vi "FlexRay_Table.vi"(8 "错误输入（无错误）":errorcluster, 9 "DataBase_array":refnum<vi>, 10 "FR_Buffer":T1[](array[typedef]), 11 "FlexRay_Data Ref":refnum<vi>) -> (0 "错误输出":errorcluster)   [LabVIEW 2014]
uses:
  Typedef/TLibFLexRay.ctl
  DataBase/Typedef/CAN/TCANSignal.ctl
  DataBase/Typedef/LIN/TLINSignal.ctl
  DataBase/Typedef/FlexRay/TFlexRaySignal.ctl
  DataBase/Typedef/TDBSignalProperties.ctl
  DataBase/Typedef/TDBFrameProperties.ctl
  DataBase/Typedef/TDBECUProperties.ctl
  DataBase/Typedef/TDBProperties.ctl
  DataBase/Typedef/DataBase_array.ctl
types:
  T1 = typedef "TLibFLexRay.ctl" = cluster{"FIdxChn":u8, "FChannelMask":u8, "FDir":u8, "FPayloadLength":u8, "FActualPayloadLength":u8, "FCycleNumber":u8, "FCCType":u8, "FFrameType":u8, "FHeaderCRCA":u16, "FHeaderCRCB":u16, "FFrameStateInfo":u16, "FSlotId":u16, "FFrameFlags":u32, "FFrameCRC":u32, "FReserved1":u64, "FReserved2":u64, "FTimeUs":u64, "FData":cluster{"数值":u8, "数值 9":u8, "数值 17":u8, "数值 25":u8, "数值 33":u8, "数值 41":u8, "数值 49":u8, "数值 57":u8, "数值 65":u8, "数值 73":u8, "数值 81":u8, "数值 89":u8, "数值 97":u8, "数值 105":u8, "数值 98":u8, "数值 99":u8, "数值 2":u8, "数值 10":u8, "数值 18":u8, "数值 26":u8, "数值 34":u8, "数值 42":u8, "数值 50":u8, "数值 58":u8, "数值 66":u8, "数值 74":u8, "数值 82":u8, "数值 90":u8, "数值 100":u8, "数值 106":u8, "数值 101":u8, "数值 102":u8, "数值 3":u8, "数值 11":u8, "数值 19":u8, "数值 27":u8, "数值 35":u8, "数值 43":u8, "数值 51":u8, "数值 59":u8, "数值 67":u8, "数值 75":u8, "数值 83":u8, "数值 91":u8, "数值 103":u8, "数值 107":u8, "数值 104":u8, "数值 108":u8, "数值 4":u8, "数值 12":u8, "数值 20":u8, "数值 28":u8, "数值 36":u8, "数值 44":u8, "数值 52":u8, "数值 60":u8, "数值 68":u8, "数值 76":u8, "数值 84":u8, "数值 92":u8, "数值 109":u8, "数值 110":u8, "数值 111":u8, "数值 112":u8, "数值 5":u8, "数值 13":u8, "数值 21":u8, "数值 29":u8, "数值 37":u8, "数值 45":u8, "数值 53":u8, "数值 61":u8, "数值 69":u8, "数值 77":u8, "数值 85":u8, "数值 93":u8, "数值 113":u8, "数值 114":u8, "数值 115":u8, "数值 116":u8, "数值 6":u8, "数值 14":u8, "数值 22":u8, "数值 30":u8, "数值 38":u8, "数值 46":u8, "数值 54":u8, "数值 62":u8, "数值 70":u8, "数值 78":u8, "数值 86":u8, "数值 94":u8, "数值 117":u8, "数值 118":u8, "数值 119":u8, "数值 120":u8, "数值 7":u8, "数值 15":u8, "数值 23":u8, "数值 31":u8, "数值 39":u8, "数值 47":u8, "数值 55":u8, "数值 63":u8, "数值 71":u8, "数值 79":u8, "数值 87":u8, "数值 95":u8, "数值 121":u8, "数值 122":u8, "数值 123":u8, "数值 124":u8, "数值 8":u8, "数值 16":u8, "数值 24":u8, "数值 32":u8, "数值 40":u8, "数值 48":u8, "数值 56":u8, "数值 64":u8, "数值 72":u8, "数值 80":u8, "数值 88":u8, "数值 96":u8, "数值 125":u8, "数值 126":u8, "数值 127":u8, "数值 128":u8, "数值 129":u8, "数值 130":u8, "数值 131":u8, "数值 132":u8, "数值 133":u8, "数值 134":u8, "数值 135":u8, "数值 136":u8, "数值 137":u8, "数值 138":u8, "数值 139":u8, "数值 140":u8, "数值 141":u8, "数值 142":u8, "数值 143":u8, "数值 144":u8, "数值 145":u8, "数值 146":u8, "数值 147":u8, "数值 148":u8, "数值 149":u8, "数值 150":u8, "数值 151":u8, "数值 152":u8, "数值 153":u8, "数值 154":u8, "数值 155":u8, "数值 156":u8, "数值 157":u8, "数值 158":u8, "数值 159":u8, "数值 160":u8, "数值 161":u8, "数值 162":u8, "数值 163":u8, "数值 164":u8, "数值 165":u8, "数值 166":u8, "数值 167":u8, "数值 168":u8, "数值 169":u8, "数值 170":u8, "数值 171":u8, "数值 172":u8, "数值 173":u8, "数值 174":u8, "数值 175":u8, "数值 176":u8, "数值 177":u8, "数值 178":u8, "数值 179":u8, "数值 180":u8, "数值 181":u8, "数值 182":u8, "数值 183":u8, "数值 184":u8, "数值 185":u8, "数值 186":u8, "数值 187":u8, "数值 188":u8, "数值 189":u8, "数值 190":u8, "数值 191":u8, "数值 192":u8, "数值 193":u8, "数值 194":u8, "数值 195":u8, "数值 196":u8, "数值 197":u8, "数值 198":u8, "数值 199":u8, "数值 200":u8, "数值 201":u8, "数值 202":u8, "数值 203":u8, "数值 204":u8, "数值 205":u8, "数值 206":u8, "数值 207":u8, "数值 208":u8, "数值 209":u8, "数值 210":u8, "数值 211":u8, "数值 212":u8, "数值 213":u8, "数值 214":u8, "数值 215":u8, "数值 216":u8, "数值 217":u8, "数值 218":u8, "数值 219":u8, "数值 220":u8, "数值 221":u8, "数值 222":u8, "数值 223":u8, "数值 224":u8, "数值 225":u8, "数值 226":u8, "数值 227":u8, "数值 228":u8, "数值 229":u8, "数值 230":u8, "数值 231":u8, "数值 232":u8, "数值 233":u8, "数值 234":u8, "数值 235":u8, "数值 236":u8, "数值 237":u8, "数值 238":u8, "数值 239":u8, "数值 241":u8, "数值 242":u8, "数值 243":u8, "数值 244":u8, "数值 245":u8, "数值 246":u8, "数值 247":u8, "数值 248":u8, "数值 249":u8, "数值 250":u8, "数值 251":u8, "数值 252":u8, "数值 253":u8, "数值 254":u8, "数值 255":u8}}
  T2 = cluster{"Message Name":string, "Signal Names":string[], "Signal_Values":dbl[]}
  T3 = cluster{"数值":u8, "数值 9":u8, "数值 17":u8, "数值 25":u8, "数值 33":u8, "数值 41":u8, "数值 49":u8, "数值 57":u8, "数值 65":u8, "数值 73":u8, "数值 81":u8, "数值 89":u8, "数值 97":u8, "数值 105":u8, "数值 98":u8, "数值 99":u8, "数值 2":u8, "数值 10":u8, "数值 18":u8, "数值 26":u8, "数值 34":u8, "数值 42":u8, "数值 50":u8, "数值 58":u8, "数值 66":u8, "数值 74":u8, "数值 82":u8, "数值 90":u8, "数值 100":u8, "数值 106":u8, "数值 101":u8, "数值 102":u8, "数值 3":u8, "数值 11":u8, "数值 19":u8, "数值 27":u8, "数值 35":u8, "数值 43":u8, "数值 51":u8, "数值 59":u8, "数值 67":u8, "数值 75":u8, "数值 83":u8, "数值 91":u8, "数值 103":u8, "数值 107":u8, "数值 104":u8, "数值 108":u8, "数值 4":u8, "数值 12":u8, "数值 20":u8, "数值 28":u8, "数值 36":u8, "数值 44":u8, "数值 52":u8, "数值 60":u8, "数值 68":u8, "数值 76":u8, "数值 84":u8, "数值 92":u8, "数值 109":u8, "数值 110":u8, "数值 111":u8, "数值 112":u8, "数值 5":u8, "数值 13":u8, "数值 21":u8, "数值 29":u8, "数值 37":u8, "数值 45":u8, "数值 53":u8, "数值 61":u8, "数值 69":u8, "数值 77":u8, "数值 85":u8, "数值 93":u8, "数值 113":u8, "数值 114":u8, "数值 115":u8, "数值 116":u8, "数值 6":u8, "数值 14":u8, "数值 22":u8, "数值 30":u8, "数值 38":u8, "数值 46":u8, "数值 54":u8, "数值 62":u8, "数值 70":u8, "数值 78":u8, "数值 86":u8, "数值 94":u8, "数值 117":u8, "数值 118":u8, "数值 119":u8, "数值 120":u8, "数值 7":u8, "数值 15":u8, "数值 23":u8, "数值 31":u8, "数值 39":u8, "数值 47":u8, "数值 55":u8, "数值 63":u8, "数值 71":u8, "数值 79":u8, "数值 87":u8, "数值 95":u8, "数值 121":u8, "数值 122":u8, "数值 123":u8, "数值 124":u8, "数值 8":u8, "数值 16":u8, "数值 24":u8, "数值 32":u8, "数值 40":u8, "数值 48":u8, "数值 56":u8, "数值 64":u8, "数值 72":u8, "数值 80":u8, "数值 88":u8, "数值 96":u8, "数值 125":u8, "数值 126":u8, "数值 127":u8, "数值 128":u8, "数值 129":u8, "数值 130":u8, "数值 131":u8, "数值 132":u8, "数值 133":u8, "数值 134":u8, "数值 135":u8, "数值 136":u8, "数值 137":u8, "数值 138":u8, "数值 139":u8, "数值 140":u8, "数值 141":u8, "数值 142":u8, "数值 143":u8, "数值 144":u8, "数值 145":u8, "数值 146":u8, "数值 147":u8, "数值 148":u8, "数值 149":u8, "数值 150":u8, "数值 151":u8, "数值 152":u8, "数值 153":u8, "数值 154":u8, "数值 155":u8, "数值 156":u8, "数值 157":u8, "数值 158":u8, "数值 159":u8, "数值 160":u8, "数值 161":u8, "数值 162":u8, "数值 163":u8, "数值 164":u8, "数值 165":u8, "数值 166":u8, "数值 167":u8, "数值 168":u8, "数值 169":u8, "数值 170":u8, "数值 171":u8, "数值 172":u8, "数值 173":u8, "数值 174":u8, "数值 175":u8, "数值 176":u8, "数值 177":u8, "数值 178":u8, "数值 179":u8, "数值 180":u8, "数值 181":u8, "数值 182":u8, "数值 183":u8, "数值 184":u8, "数值 185":u8, "数值 186":u8, "数值 187":u8, "数值 188":u8, "数值 189":u8, "数值 190":u8, "数值 191":u8, "数值 192":u8, "数值 193":u8, "数值 194":u8, "数值 195":u8, "数值 196":u8, "数值 197":u8, "数值 198":u8, "数值 199":u8, "数值 200":u8, "数值 201":u8, "数值 202":u8, "数值 203":u8, "数值 204":u8, "数值 205":u8, "数值 206":u8, "数值 207":u8, "数值 208":u8, "数值 209":u8, "数值 210":u8, "数值 211":u8, "数值 212":u8, "数值 213":u8, "数值 214":u8, "数值 215":u8, "数值 216":u8, "数值 217":u8, "数值 218":u8, "数值 219":u8, "数值 220":u8, "数值 221":u8, "数值 222":u8, "数值 223":u8, "数值 224":u8, "数值 225":u8, "数值 226":u8, "数值 227":u8, "数值 228":u8, "数值 229":u8, "数值 230":u8, "数值 231":u8, "数值 232":u8, "数值 233":u8, "数值 234":u8, "数值 235":u8, "数值 236":u8, "数值 237":u8, "数值 238":u8, "数值 239":u8, "数值 241":u8, "数值 242":u8, "数值 243":u8, "数值 244":u8, "数值 245":u8, "数值 246":u8, "数值 247":u8, "数值 248":u8, "数值 249":u8, "数值 250":u8, "数值 251":u8, "数值 252":u8, "数值 253":u8, "数值 254":u8, "数值 255":u8}
  T4 = typedef "LVRowAndColumnUnsignedTypeDef.ctl" = cluster{"Row":u32, "Column":u32}
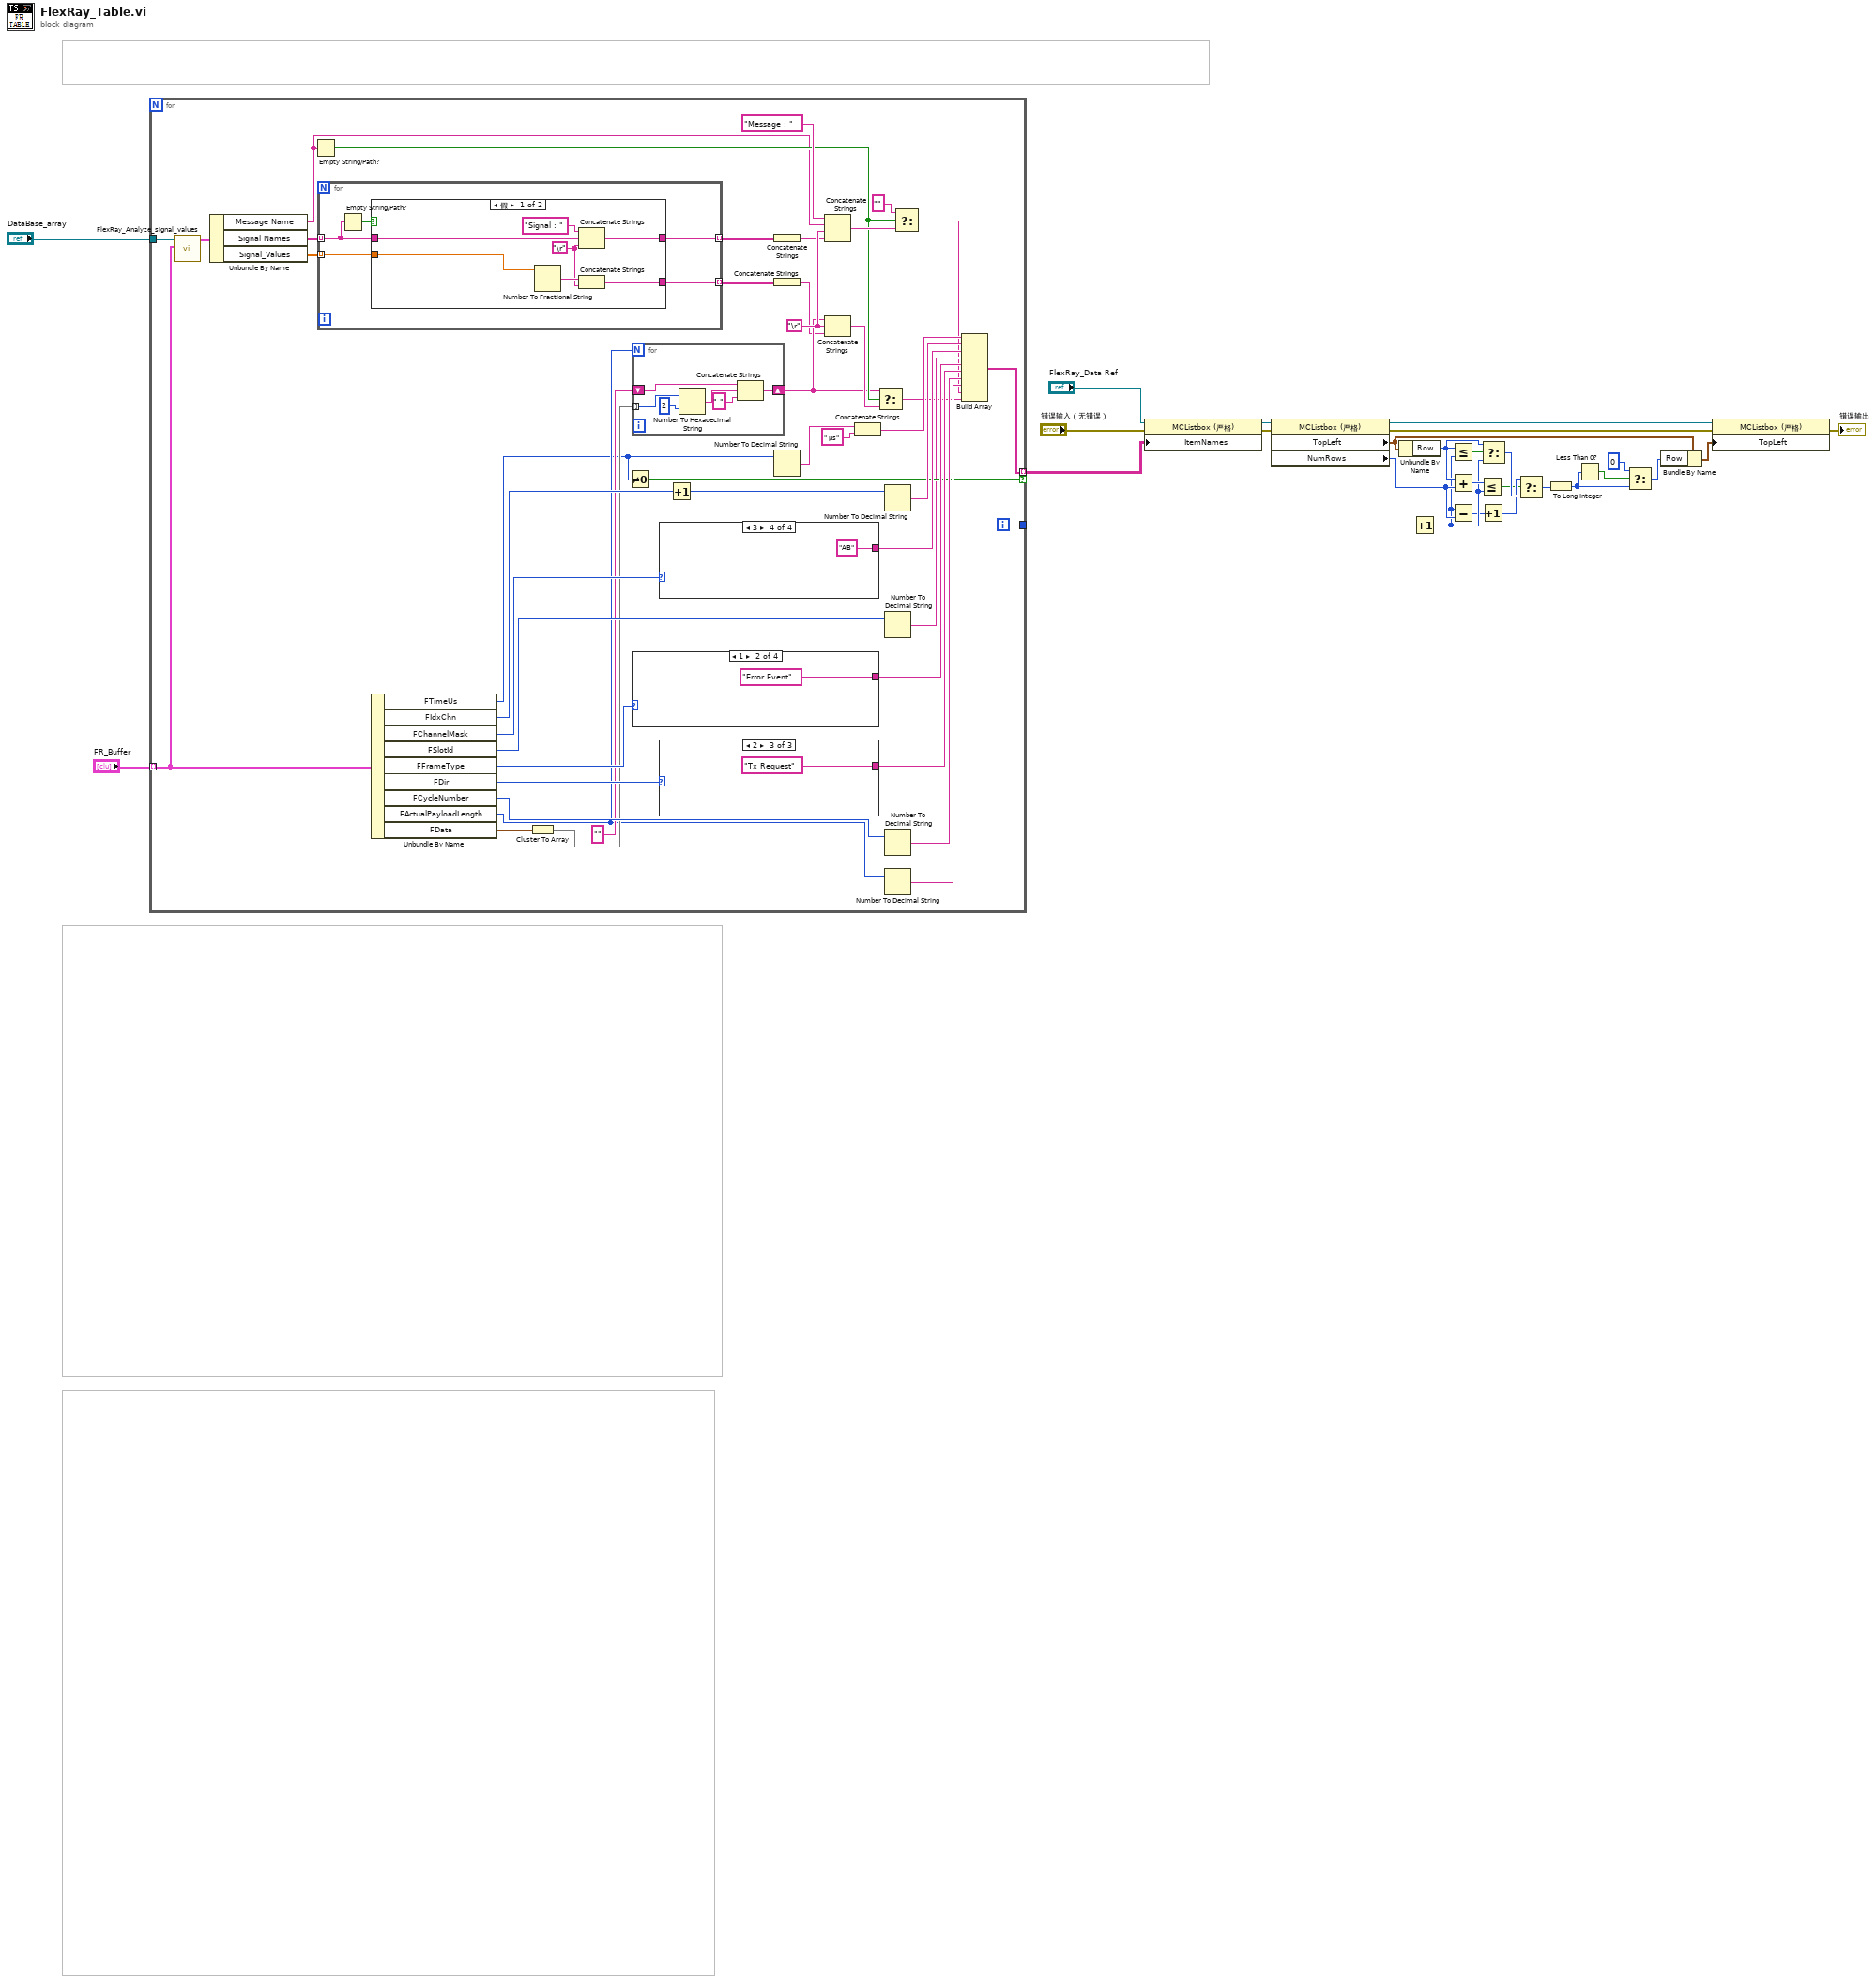
[diagram p0: block diagram]
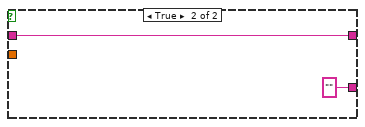
[diagram p2: hidden frame]
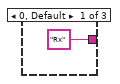
[diagram p3: hidden frame]
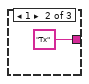
[diagram p4: hidden frame]
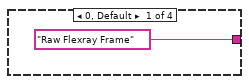
[diagram p5: hidden frame]
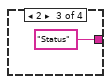
[diagram p6: hidden frame]
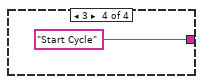
[diagram p7: hidden frame]
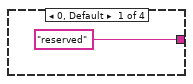
[diagram p8: hidden frame]
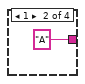
[diagram p9: hidden frame]
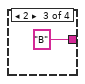
[diagram p10: hidden frame]
diagram:
  n1 = for {
    tunnel: "FR_Buffer" -> [w45] mode=indexing
    tunnel: [w51] -> w3 mode=indexing if=w48
    tunnel: [w50] -> w2
    tunnel: "DataBase_array" -> [w46]
    i -> [w50]
    w35 = "\r"
    n2 = call "FlexRay_Analyze_signal_values.vi"("TLibFLexRay"=w45, "DataBase_array"=w46) -> ("data out"=w44:T2)  [unwired: 9 in]
    n3 = Unbundle By Name(w44) -> ("Message Name"=w32:string, "Signal Names"=w41:string[], "Signal_Values"=w40:dbl[])
    n4 = Empty String/Path?(string/path=w32) -> (empty?=w34:bool)
    n5 = for {
      tunnel: w41 -> [w76] mode=indexing
      tunnel: [w75] -> w43 mode=indexing
      tunnel: w40 -> [w73] mode=indexing
      tunnel: [w72] -> w42 mode=indexing
      n6 = Empty String/Path?(string/path=w76) -> (empty?=w74:bool)
      n7 = case shown="假" w74 {
        tunnel: w76 -> [w83 w85]
        tunnel: [w82 w85] -> w75
        tunnel: w73 -> [w80 _]
        tunnel: [w77 ""] -> w72
        frame False {
          w78 = "\r"
          n8 = Number To Fractional String(number=w80) -> (F-format string=w79:string)  [unwired: 3 in]
          n9 = Concatenate Strings("Signal : " ("字符串"), w83, w78) -> (w82:string)
          n10 = Concatenate Strings(w79, w78) -> (w77:string)
        }
        frame True {
        }
      }
    }
    n11 = Unbundle By Name(w45) -> ("FTimeUs"=w49:u64, "FIdxChn"=w67:u8, "FChannelMask"=w65:u8, "FSlotId"=w63:u16, "FFrameType"=w62:u8, "FDir"=w60:u8, "FCycleNumber"=w58:u8, "FActualPayloadLength"=w52:u8, "FData"=w54:T3)
    n12 = Cluster To Array(cluster=w54) -> (array=w53:u8[])
    n13 = Not Equal To 0?(x=w49) -> (x != 0?=w48:bool)
    n14 = for {
      N: w52 -> [_]
      shift-right: [w90] -> w30
      shift-left: "" -> [w91]
      tunnel: w53 -> [w86] mode=indexing
      n15 = Number To Hexadecimal String(1:i16 2 ("width (-)"), 2:w86) -> (0:w88:string)
      n16 = Concatenate Strings(w91, w88, " " ("string")) -> (w90:string)
    }
    n17 = case shown="1" w62 {
      tunnel: ["Raw Flexray Frame" "Error Event" "Status" "Start Cycle"] -> w61
      frame 0, Default {
      }
      frame 1 {
      }
      frame 2 {
      }
      frame 3 {
      }
    }
    n18 = case shown="3" w65 {
      tunnel: ["reserved" "A" "B" "AB"] -> w64
      frame 0, Default {
      }
      frame 1 {
      }
      frame 2 {
      }
      frame 3 {
      }
    }
    n19 = case shown="2" w60 {
      tunnel: ["Rx" "Tx" "Tx Request"] -> w59
      frame 0, Default {
      }
      frame 1 {
      }
      frame 2 {
      }
    }
    n20 = Increment(x=w67) -> (x+1=w68:u8)
    n21 = Concatenate Strings(w43) -> (w31:string)
    n22 = Concatenate Strings(w42) -> (w29:string)
    n23 = Number To Decimal String(number=w49) -> (decimal integer string=w70:string)  [unwired: 1 in]
    n24 = Concatenate Strings("Message : " ("字符串"), w32, w35, w31) -> (w38:string)
    n25 = Concatenate Strings(w30, w35, w29) -> (w37:string)
    n26 = Concatenate Strings(w70, " μs" ("字符串")) -> (w69:string)
    n27 = Select(t=w30, s=w34, f=w37) -> (s? t:f=w28:string)
    n28 = Number To Decimal String(number=w68) -> (decimal integer string=w66:string)  [unwired: 1 in]
    n29 = Number To Decimal String(number=w63) -> (decimal integer string=w47:string)  [unwired: 1 in]
    n30 = Number To Decimal String(number=w58) -> (decimal integer string=w57:string)  [unwired: 1 in]
    n31 = Number To Decimal String(number=w52) -> (decimal integer string=w56:string)  [unwired: 1 in]
    n32 = Select(t="", s=w34, f=w38) -> (s? t:f=w33:string)
    n33 = Build Array(w69, w66, w64, w47, w61, w59, w57, w56, w33, w28) -> (w51:string[])
  }
  n34 = property class="MCListbox (严格)"(reference="FlexRay_Data Ref", error in="错误输入（无错误）", "ItemNames"=w3) -> (reference out=w10:refnum<vi>, error out=w8:errorcluster)
  n35 = property class="MCListbox (严格)"(reference=w10, error in=w8) -> (reference out=w18:refnum<vi>, error out=w7:errorcluster, "TopLeft"=w17:T4, "NumRows"=w25:u32)
  n36 = Unbundle By Name(w17) -> ("Row"=w26:u32)
  n37 = Increment(x=w2) -> (x+1=w23:i32)
  n38 = Less Or Equal?(x=w26, y=w23) -> (x <= y?=w27:bool)
  n39 = Add(x=w26, y=w25) -> (x+y=w24:u32)
  n40 = Subtract(x=w23, y=w25) -> (x-y=w22:u32)
  n41 = Less Or Equal?(x=w24, y=w23) -> (x <= y?=w19:bool)
  n42 = Increment(x=w22) -> (x+1=w20:u32)
  n43 = Select(t=w26, s=w27, f=w23) -> (s? t:f=w21:u32)
  n44 = Select(t=w20, s=w19, f=w21) -> (s? t:f=w16:u32)
  n45 = To Long Integer(number=w16) -> (32bit integer=w14:i32)
  n46 = Less Than 0?(x=w14) -> (x < 0?=w15:bool)
  n47 = Select(t=0, s=w15, f=w14) -> (s? t:f=w13:i32)
  n48 = Bundle By Name(cluster=w17, "Row"=w13) -> (w11:T4)
  n49 = property class="MCListbox (严格)"(reference=w18, error in=w7, "TopLeft"=w11) -> (error out=→"错误输出":errorcluster)  [unwired: 1 out]
